vi "GetSystemPowerStatus Kernel32 dll.vi"() -> (2 "BatteryLifePercent":u8)   [LabVIEW 2025]
doc: "This example demonstrates how to use a Call Library Function Node to call the GetSystemInfo function. The GetSystemInfo function returns information about the current system, such as number of processors and processor type.\n\nNote: To retrieve accurate information for a Win32-based application running on WOW64 (Windows-on-Windows 64-bit), call the GetNativeSystemInfo function. For more information about the call setup, refer to the GetNativeSystemInfo topic on the MSDN Web site.\n\nThe block diagram includes information about the values returned by the function call. These values are defined in the GetSystemInfo topic on the MSDN Web site."
uses:
  kernel32.dll
panel:
  out "sysinfo":T1
  # "Select Help»Show Context Help and move the cursor\nover the VI icon to display help for this VI."
  # "http://msdn.microsoft.com/en-us/library/aa372693(VS.85).aspx"
  # "http://msdn.microsoft.com/en-us/library/aa373232(VS.85).aspx"
  # "typedef struct _SYSTEM_POWER_STATUS {\n  BYTE  ACLineStatus;\n  BYTE  BatteryFlag;\n  BYTE  BatteryLifePercent;\n  BYTE  Reserved1;\n  DWORD BatteryLifeTime;\n  DWORD BatteryFullLifeTime;\n}SYSTEM_POWER_STATUS, *LPSYSTEM_POWER_STATUS;"
  # "Members\nACLineStatus \nThe AC power status. This member can be one of the following values. \n0 Offline\n1 Online\n255 Unknown status\n \nBatteryFlag \nThe battery charge status. This member can contain one or more of the following flags. \n\nValue Meaning \n1 High—the battery capacity is at more than 66 percent\n 2 Low—the battery capacity is at less than 33 percent\n 4 Critical—the battery capacity is at less than five percent\n 8 Charging\n 128 No system battery\n 255 Unknown status—unable to read the battery flag information\nThe value is zero if the battery is not being charged and the battery capacity is between low and high.\n\nBatteryLifePercent \nThe percentage of full battery charge remaining. This member can be a value in the range 0 to 100, or 255 if status is unknown.\n\nReserved1 \nReserved; must be zero.\n\nBatteryLifeTime \nThe number of seconds of battery life remaining, or –1 if remaining seconds are unknown.\n\nBatteryFullLifeTime \nThe number of seconds of battery life when at full charge, or –1 if full battery lifetime is unknown.\n\nRemarks\nThe system is only capable of estimating BatteryFullLifeTime based on calculations on BatteryLifeTime and BatteryLifePercent. Without smart battery subsystems, this value may not be accurate enough to be useful."
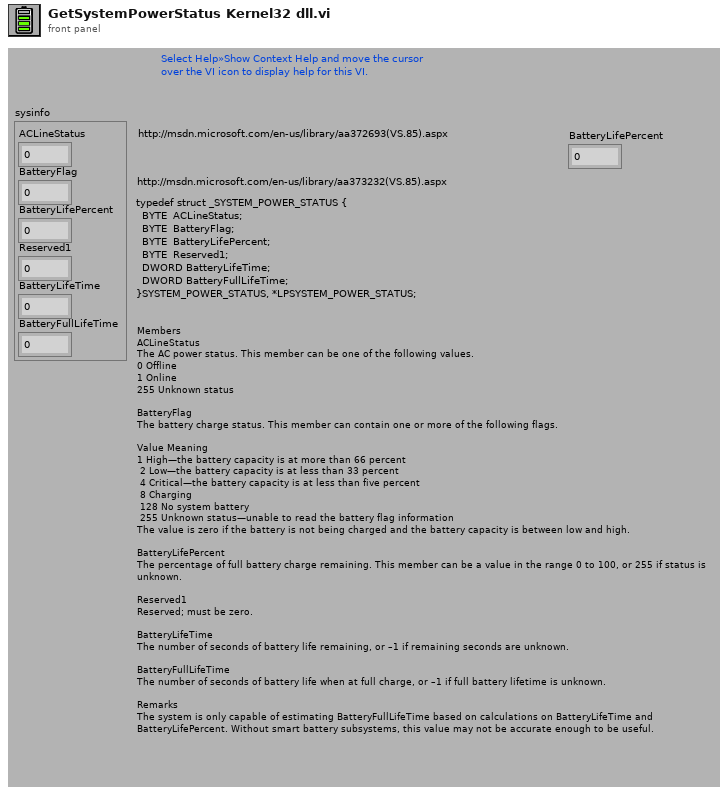
[diagram p1: front panel]
types:
  T1 = cluster{"ACLineStatus":u8, "BatteryFlag":u8, "BatteryLifePercent":u8, "Reserved1":u8, "BatteryLifeTime":u32, "BatteryFullLifeTime":u32}
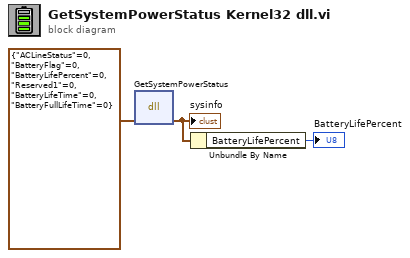
[diagram p0: block diagram]
diagram:
  n1 = dll-call lib="KERNEL32.DLL" fn="GetSystemPowerStatus"("sysinfo"=T1 {"ACLineStatus"=0, "BatteryFlag"=0, "BatteryLifePercent"=0, "Reserved1"=0, "BatteryLifeTime"=0, "BatteryFullLifeTime"=0}) -> ("sysinfo"=w2:T1)  [unwired: 3 in, 3 out]
  "sysinfo" <- w2
  n2 = Unbundle By Name(w2) -> ("BatteryLifePercent"=→"BatteryLifePercent":u8)
